vi "SortableDateTimes.vi"(11 "seconds since 1Jan1904":timestamp) -> (3 "SortableDate-Times":string)   [LabVIEW 2015]
uses:
  <vilib>/Utility/miscctls.llb/LVDateTimeRec.ctl
panel:
  out "SecondsSinceMidnight":dbl
  out "DayOfMonth":string
  out "Month":string
  out "DayOfWeek":string
  out "DayName":string
  out "Year":string
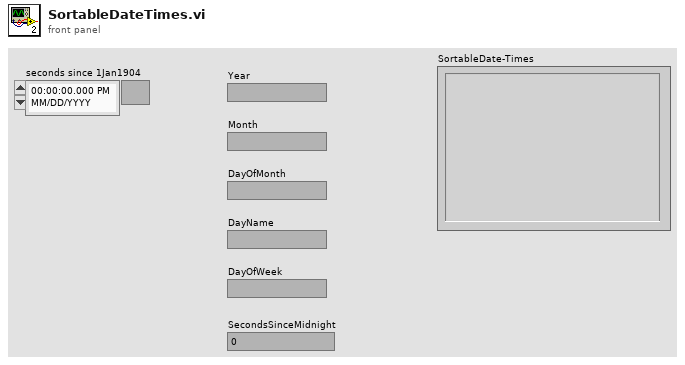
[diagram p1: front panel]
types:
  T1 = typedef "LVDateTimeRec.ctl" = cluster{"fractional second":dbl, "second":i32, "minute":i32, "hour":i32, "day of month":i32, "month":i32, "year":i32, "day of week":i32, "day of year":i32, "DST":i32}
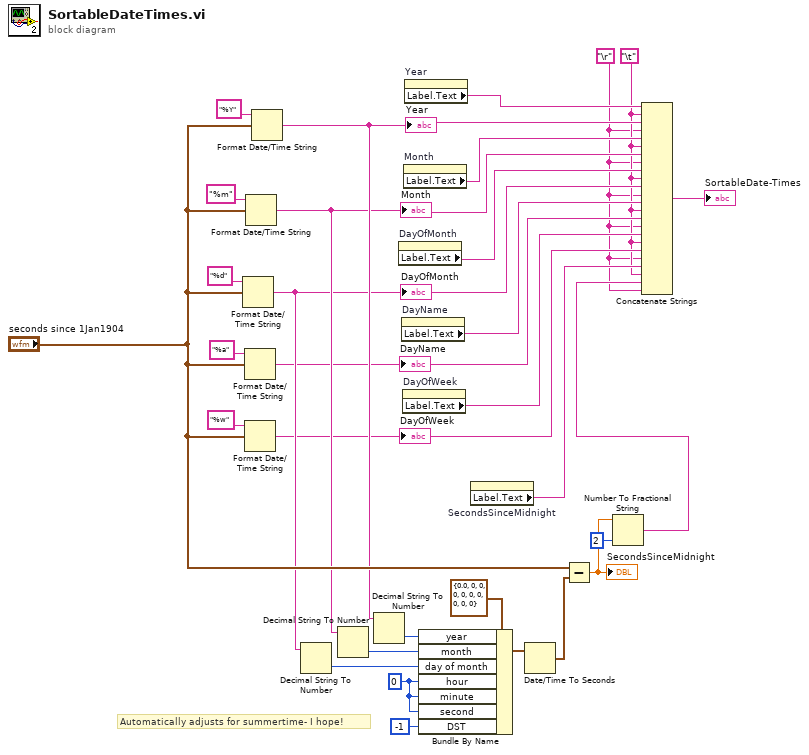
[diagram p0: block diagram]
diagram:
  w1 = "\r"
  w3 = "\t"
  w29 = 0 ("hour")
  # "Automatically adjusts for summertime- I hope!"
  n1 = Format Date/Time String(time format string (%c)="%d", seconds (now)="seconds since 1Jan1904") -> (date/time string=w11:string)  [unwired: 1 in]
  "DayOfMonth" <- w11
  n2 = Format Date/Time String(time format string (%c)="%a", seconds (now)="seconds since 1Jan1904") -> (date/time string=w9:string)  [unwired: 1 in]
  "DayName" <- w9
  n3 = Format Date/Time String(time format string (%c)="%w", seconds (now)="seconds since 1Jan1904") -> (date/time string=w7:string)  [unwired: 1 in]
  "DayOfWeek" <- w7
  n4 = Format Date/Time String(time format string (%c)="%m", seconds (now)="seconds since 1Jan1904") -> (date/time string=w13:string)  [unwired: 1 in]
  "Month" <- w13
  n5 = Format Date/Time String(time format string (%c)="%Y", seconds (now)="seconds since 1Jan1904") -> (date/time string=w16:string)  [unwired: 1 in]
  "Year" <- w16
  n6 = Decimal String To Number(string=w11) -> (number=w27:i32)  [unwired: 2 in, 1 out]
  n7 = Decimal String To Number(string=w13) -> (number=w26:i32)  [unwired: 2 in, 1 out]
  n8 = Decimal String To Number(string=w16) -> (number=w25:i32)  [unwired: 2 in, 1 out]
  n9 = property on="DayOfMonth" class="Str"() -> ("Label.Text"=w12:string)  [unwired: 2 in, 2 out]
  n10 = property on="DayName" class="Str"() -> ("Label.Text"=w10:string)  [unwired: 2 in, 2 out]
  n11 = property on="DayOfWeek" class="Str"() -> ("Label.Text"=w8:string)  [unwired: 2 in, 2 out]
  n12 = property on="Month" class="Str"() -> ("Label.Text"=w14:string)  [unwired: 2 in, 2 out]
  n13 = property on="Year" class="Str"() -> ("Label.Text"=w17:string)  [unwired: 2 in, 2 out]
  n14 = Bundle By Name(cluster=T1 {"fractional second"=0.0, "second"=0, "minute"=0, "hour"=0, "day of month"=0, "month"=0, "year"=0, "day of week"=0, "day of year"=0, "DST"=0} ("date time rec"), "year"=w25, "month"=w26, "day of month"=w27, "hour"=w29, "minute"=w29, "second"=w29, "DST"=-1) -> (w23:T1)
  n15 = property on="SecondsSinceMidnight" class="DigNum (strict)"() -> ("Label.Text"=w4:string)  [unwired: 2 in, 2 out]
  n16 = Date/Time To Seconds(2:w23) -> (0:w28:timestamp)  [unwired: 1 in]
  n17 = Subtract(x="seconds since 1Jan1904", y=w28) -> (x-y=w6:dbl)
  "SecondsSinceMidnight" <- w6
  n18 = Number To Fractional String(number=w6, precision (6)=i16 2) -> (F-format string=w2:string)  [unwired: 2 in]
  n19 = Concatenate Strings(w17, w3, w16, w1, w14, w3, w13, w1, w12, w3, w11, w1, w10, w3, w9, w1, w8, w3, w7, w1, w4, w3, w2, w1) -> (→"SortableDate-Times":string)
